vi "BM_mcDAQ_DIO_SubVI.vi"(8 "BoardNum":u32, 10 "BitValue":bool, 11 "BitNum":u32=4) -> (3 "Control out":bool)   [LabVIEW 2021]
uses:
  <vilib>/ULx/Create Channel.llb/ULx Create Channel (DO-Digital Output).vi
  <vilib>/ULx/Write.llb/ULx Write (Digital Bool 1Line 1Point).vi
panel:
  out "error out":errorcluster
  # "PeTeR\n\nBoard: #1 (Configure using InstaCal)\n\nBit Numbers:\n0 = Sparging\n2 = Cool Trap\n4 = Drying Flow\n5 = Valve Position A\n6 = Valve Position B\n7 = Heat Trap"
  # "OSSCAR\n\nBoard: #0 (Configure using InstaCal)\n\nBit Numbers:\n0 = Sparging\n1 = Valve Position A\n2 = Valve Position B\n3 = EC vent\n4 = Cool Trap\n5 = Sparge Dir\n6 = Sample Dir\n7 = Heat Trap"
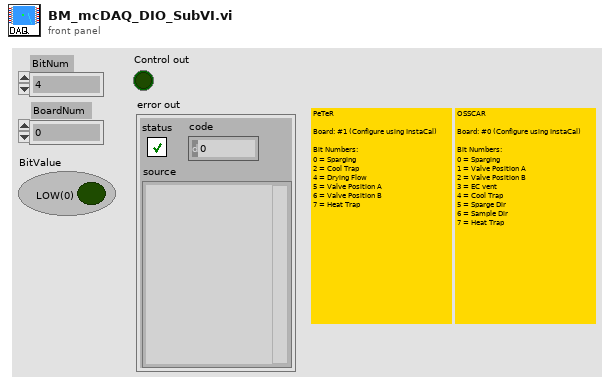
[diagram p1: front panel]
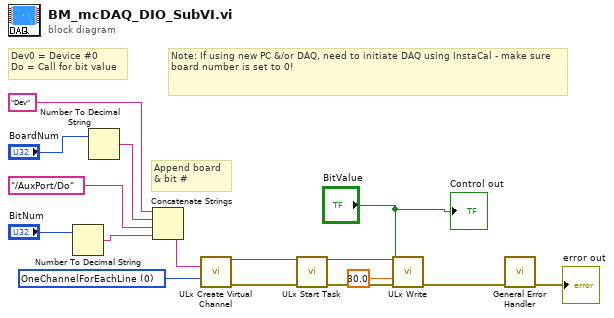
[diagram p0: block diagram]
diagram:
  w16 = 0 items=["OneChannelForEachLine", "OneChannelForAllLines"] ("line grouping")
  # "Note: If using new PC &/or DAQ, need to initiate DAQ using InstaCal - make sure board number is set to 0!"
  # "Append board\n& bit #"
  # "Dev0 = Device #0\nDo = Call for bit value"
  n1 = Number To Decimal String(number="BitNum") -> (decimal integer string=w6:string)  [unwired: 1 in]
  n2 = Number To Decimal String(number="BoardNum") -> (decimal integer string=w4:string)  [unwired: 1 in]
  n3 = Concatenate Strings("Dev", w4, "/AuxPort/Do", w6) -> (w12:string)
  n4 = call-poly <vilib>:"ULx Create Virtual Channel.vi"("lines"=w12, "line grouping"=w16) -> ("task out"=w15:refnum<k24>, "error out"=w11:errorcluster)  [unwired: 12 in]
  n5 = call <vilib>:"ULx Start Task.vi"("task in"=w15, "error in"=w11) -> ("task out"=w14:refnum<k24>, "error out"=w10:errorcluster)  [unwired: 12 in]
  n6 = call-poly <vilib>:"ULx Write.vi"("task in"=w14, "data"="BitValue", "timeout"=30.0, "error in"=w10) -> ("error out"=w9:errorcluster)  [unwired: 9 in, 2 out]
  n7 = call <vilib>:"General Error Handler.vi"("error in (no error)"=w9) -> ("error out"=→"error out":errorcluster)  [unwired: 10 in, 4 out]
  "Control out" <- "BitValue"
